vi "Undeploy Stimulus Profile Session.vi"(8 "error in (no error)":errorcluster, 11 "Session Ref in":T1) -> (0 "error out":errorcluster, 3 "Session Ref out":T1)   [LabVIEW 2020, in "NI_VS Sequence Execution Interface.lvlib"]
doc: "Undeploys the stimulus profile session. Undeploying a session removes all data from that session and from any targets, and immediately terminates any running sequences."
uses:
  <vilib>/NI VeriStand/Execution/SequenceExecutionInterface/NI_VS Sequence Execution Interface.lvlib
  <vilib>/NI VeriStand/Execution/SequenceExecutionInterface/Stimulus Profile Session Ref.ctl
  NationalInstruments.VeriStand.ClientAPI
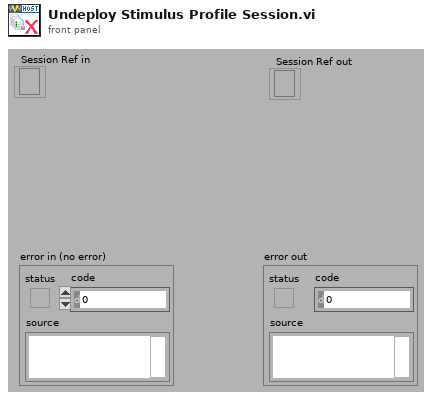
[diagram p1: front panel]
types:
  T1 = typedef "NI_VS Sequence Execution Interface.lvlib/Stimulus Profile Session Ref.ctl" = refnum<k24>
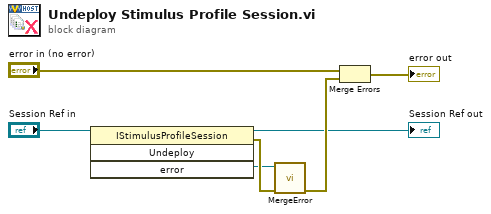
[diagram p0: block diagram]
diagram:
  n1 = invoke class="IStimulusProfileSession" method="Undeploy"(reference="Session Ref in") -> (reference out=→"Session Ref out":T1, error out=w4:errorcluster, "error"=w1:refnum<k24>)  [unwired: 3 in, 1 out]
  n2 = call <vilib>:"MergeError.vi"("error in (no error)"=w4, "Error"=w1) -> ("error out"=w3:errorcluster)  [unwired: 9 out]
  n3 = Merge Errors("error in (no error)", w3) -> (→"error out":errorcluster)
